vi "Tab-Control.vi"() -> ()   [LabVIEW 2014]
panel:
  in  "disable":bool
  in  "stop":bool
  in  "Tab Control":enum32{"Page 1", "Page 2"}(tab)
  # "Page 2 disable"
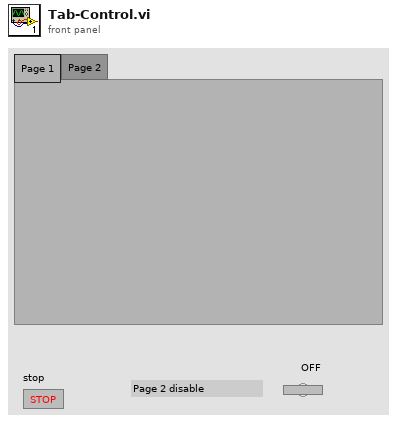
[diagram p1: front panel]
types:
  T1 = enum32{"Page Enabled", "Page Disabled", "Page Disabled & Grayed"}
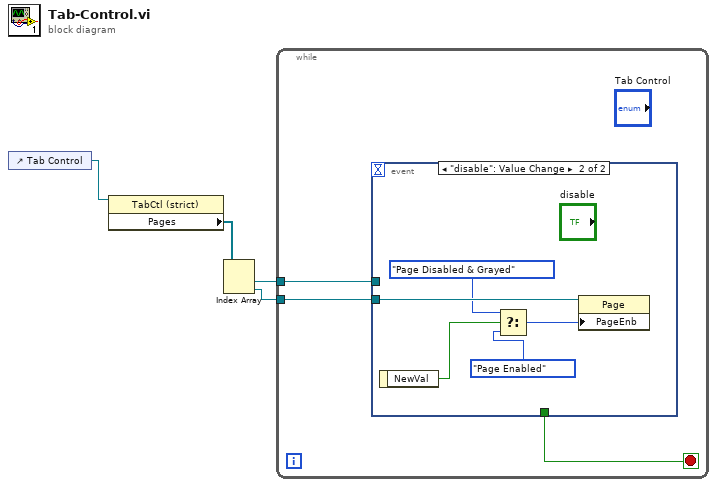
[diagram p0: block diagram]
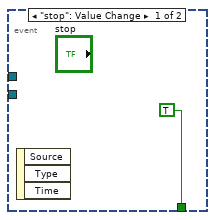
[diagram p2: hidden frame]
diagram:
  n1 = control-ref of="Tab Control"() -> (w4:refnum<vi>)
  n2 = property class="TabCtl (strict)"(reference=w4) -> ("Pages"=w3:refnum<vi>[])  [unwired: 1 in, 2 out]
  n3 = Index Array(array=w3) -> (element #1=w2:refnum<vi>, element #2=w1:refnum<vi>)  [unwired: 2 in]
  n4 = while {
    tunnel: w2 -> [w7]
    tunnel: w1 -> [w6]
    stop <- w5 stop-if-true
    n5 = event shown="[1] \"disable\": Value Change" {
      selector: _ -> [_ _]
      dyn-events: _ -> [_ _]
      timeout: _ -> [_ _]
      tunnel: w7 -> [_ _]
      tunnel: w6 -> [_ w12]
      tunnel: [TRUE _] -> w5
      event "stop": Value Change {
        n6 = event-data() -> ()  [unwired: 1 in, 3 out]
      }
      event "disable": Value Change {
        n7 = event-data() -> ("NewVal"=w13:bool)  [unwired: 1 in]
        n8 = Select(t=T1."Page Disabled & Grayed" ("Page Enabled State"), s=w13, f=T1."Page Enabled" ("Page Enabled State")) -> (s? t:f=w9:T1)
        n9 = property class="Page"(reference=w12, "PageEnb"=w9) -> ()  [unwired: 1 in, 2 out]
      }
    }
  }
